vi "FIR Filter.vi"(0 "stream in":T1, 2 "decimation factor (1)":i32=1, 3 "filter coefficients":dbl[](array[numeric]) format="%.2f", 4 "interpolation factor (1)":i32=1) -> (1 "stream out":T1)   [LabVIEW 2023]
doc: "This VI implements an FIR filter, reading data from an input Stream Channel and writing filtered data at a different rate to an output Stream Channel."
uses:
  <extravilib>/ChannelInstances/Stream-dbl/)Channel.ctl
  <extravilib>/ChannelInstances/Stream-dbl/Read With Abort.vi
  <extravilib>/ChannelInstances/Stream-dbl/Write With Abort.vi
  <extravilib>/ChannelInstances/Stream-dbl/EndpointRead.vi
  <extravilib>/ChannelInstances/Stream-dbl/Endpoint.vi
  <extravilib>/ChannelInstances/Stream-dbl/)Channel.vi
  <resource>/ChannelSupport/_ChannelSupport/WaitIfNeeded.vi
  <extravilib>/ChannelInstances/Stream-dbl.lvlib
panel:
  out "output value":dbl
  out "input value":dbl
  out "filter bank":dbl[][](array[numeric]) format="%.2f"
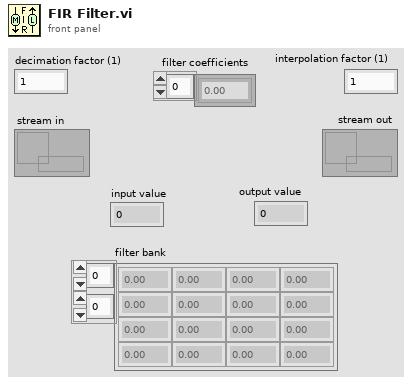
[diagram p1: front panel]
types:
  T1 = typedef "Stream-dbl.lvlib/)Channel.ctl" = refnum<queue>
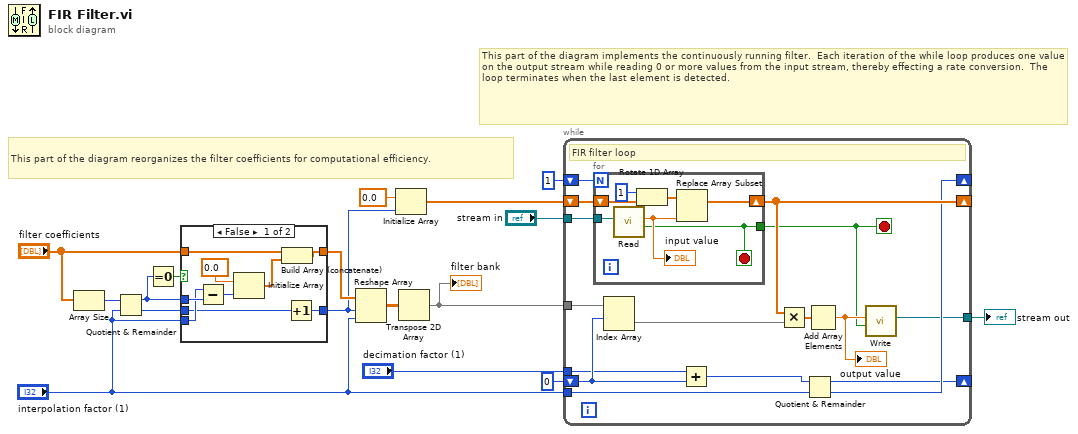
[diagram p0: block diagram]
diagram:
  # "This part of the diagram implements the continuously running filter.  Each iteration of the while loop produces one value on the output stream while reading 0 or more values from the input stream, thereby effecting a rate conversion.  The loop terminates when the last element is detected."
  # "This part of the diagram reorganizes the filter coefficients for computational efficiency."
  n1 = Array Size(array="filter coefficients") -> (size(s)=w13:i32)
  n2 = Quotient & Remainder(x=w13, y="interpolation factor (1)") -> (x-y*floor(x/y)=w9:i32, floor(x/y)=w8:i32)
  n3 = Equal To 0?(x=w9) -> (x = 0?=w12:bool)
  n4 = case shown="False" w12 {
    tunnel: "filter coefficients" -> [w19 w28]
    tunnel: [w20 w28] -> w10
    tunnel: w9 -> [w26 _]
    tunnel: "interpolation factor (1)" -> [w25 _]
    tunnel: [w23 w27] -> w5
    tunnel: w8 -> [w24 w27]
    frame False {
      n5 = Subtract(x=w25, y=w26) -> (x-y=w22:i32)
      n6 = Initialize Array(0.0 ("element"), w22) -> (w18:dbl[])
      n7 = Build Array (concatenate)(w19, w18) -> (w20:dbl[])
      n8 = Increment(x=w24) -> (x+1=w23:i32)
    }
    frame True {
    }
  }
  n9 = Reshape Array(w10, w5, "interpolation factor (1)") -> (w7:dbl[][])
  n10 = Initialize Array(0.0 ("element"), w5) -> (w16:dbl[])
  n11 = Transpose 2D Array(2D array=w7) -> (transposed array=w4:dbl[][])
  "filter bank" <- w4
  n12 = while {
    shift-right: [w38] -> _
    shift-left: w16 -> [w37]
    shift-right: [w34] -> _
    shift-left: 0 -> [w41]
    tunnel: w4 -> [w44]
    shift-right: [w35] -> _
    shift-left: 1 -> [w36]
    tunnel: "interpolation factor (1)" -> [w39]
    tunnel: "stream in" -> [w33]
    tunnel: [w30] -> w2
    tunnel: "decimation factor (1)" -> [w29]
    stop <- w31 stop-if-true
    # "FIR filter loop"
    n13 = for {
      N: w36 -> [_]
      shift-right: [w50] -> w38
      shift-left: w37 -> [w49]
      tunnel: w33 -> [w47]
      tunnel: [w45] -> w31
      stop <- w45 stop-if-true
      n14 = call <extravilib>:"Read.vi"("channel"=w47) -> ("last element?"=w45:bool, "element"=w46:dbl)  [unwired: 6 in, 3 out]
      "input value" <- w46
      n15 = Rotate 1D Array(1:w49, 2:1 ("n")) -> (0:w51:dbl[])
      n16 = Replace Array Subset(array=w51, new element=w46) -> (w50:dbl[])  [unwired: 1 in]
    }
    n17 = Index Array(array=w44, index (row)=w41) -> (element=w43:dbl[])  [unwired: 1 in]
    n18 = Add(x=w29, y=w41) -> (x+y=w40:i32)
    n19 = Multiply(x=w38, y=w43) -> (x*y=w42:dbl[])
    n20 = Quotient & Remainder(x=w40, y=w39) -> (x-y*floor(x/y)=w34:i32, floor(x/y)=w35:i32)
    n21 = Add Array Elements(numeric array=w42) -> (sum=w32:dbl)
    "output value" <- w32
    n22 = call <extravilib>:"Write.vi"("last element? (F)"=w31, "element"=w32) -> ("channel"=w30:T1)  [unwired: 7 in, 2 out]
  }
  "stream out" <- w2
